vi "2019-05-013_FormulaNode_01.vi"() -> ()   [LabVIEW 2018]
panel:
  out "z":dbl
  in  "y":dbl
  in  "x":dbl
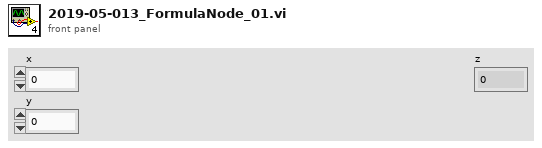
[diagram p1: front panel]
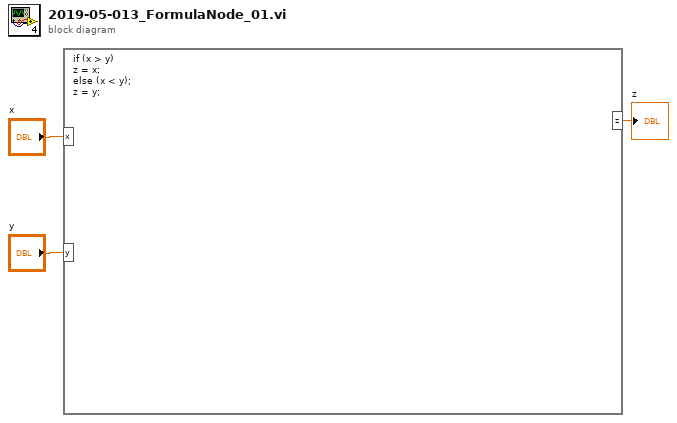
[diagram p0: block diagram]
diagram:
  n1 = formula code="if (x > y)\nz = x;\nelse (x < y);\nz = y;"("x"="x", "y"="y") -> ("z"=→"z":dbl)
